vi "initiate.vi"(8 "error in (no error)":errorcluster, 11 "reference in":refnum<class "Devices Controller.lvclass">) -> (0 "error out":errorcluster, 3 "reference out":refnum<class "Devices Controller.lvclass">)   [LabVIEW 2016, in "Devices Controller.lvclass"]
uses:
  Devices Controller.lvclass
  File Controller_llb/File Controller.lvclass
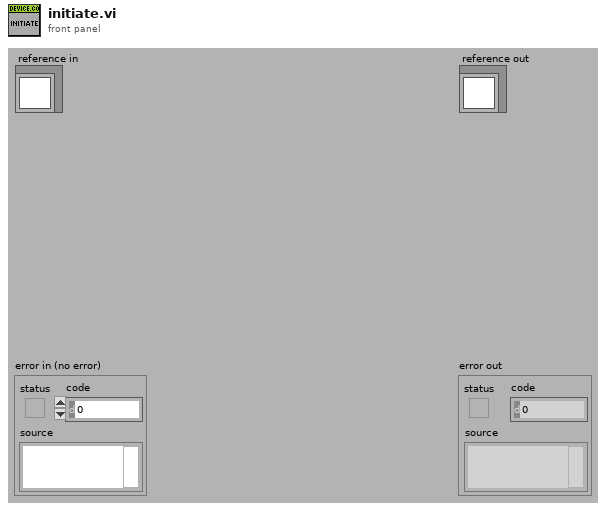
[diagram p1: front panel]
types:
  T1 = typedef "Devices Controller.lvclass/ObjectAttributesRef.ctl" = refnum<data-value>
  T2 = typedef "Devices Controller.lvclass/ObjectAttributes.ctl" = cluster{"MyAttribute":dbl, "file_controller_ref":refnum<class "File Controller.lvclass">, "data":string[][][], "devices_refs":cluster{"k4b2_refs":refnum<class "k4b2.lvclass">[], "rmr_refs":refnum<class "rmr.lvclass">[], "bod_pod_refs":refnum<class "bodpod.lvclass">[], "cpet_refs":refnum<class "cpet.lvclass">[], "fitmate_refs":refnum<class "fitmate.lvclass">[], "pea_pod_refs":refnum<class "peapod.lvclass">[], "k5_refs":refnum<class "k5.lvclass">[], "bb-pft_refs":refnum<class "bb-pft.lvclass">[]}}
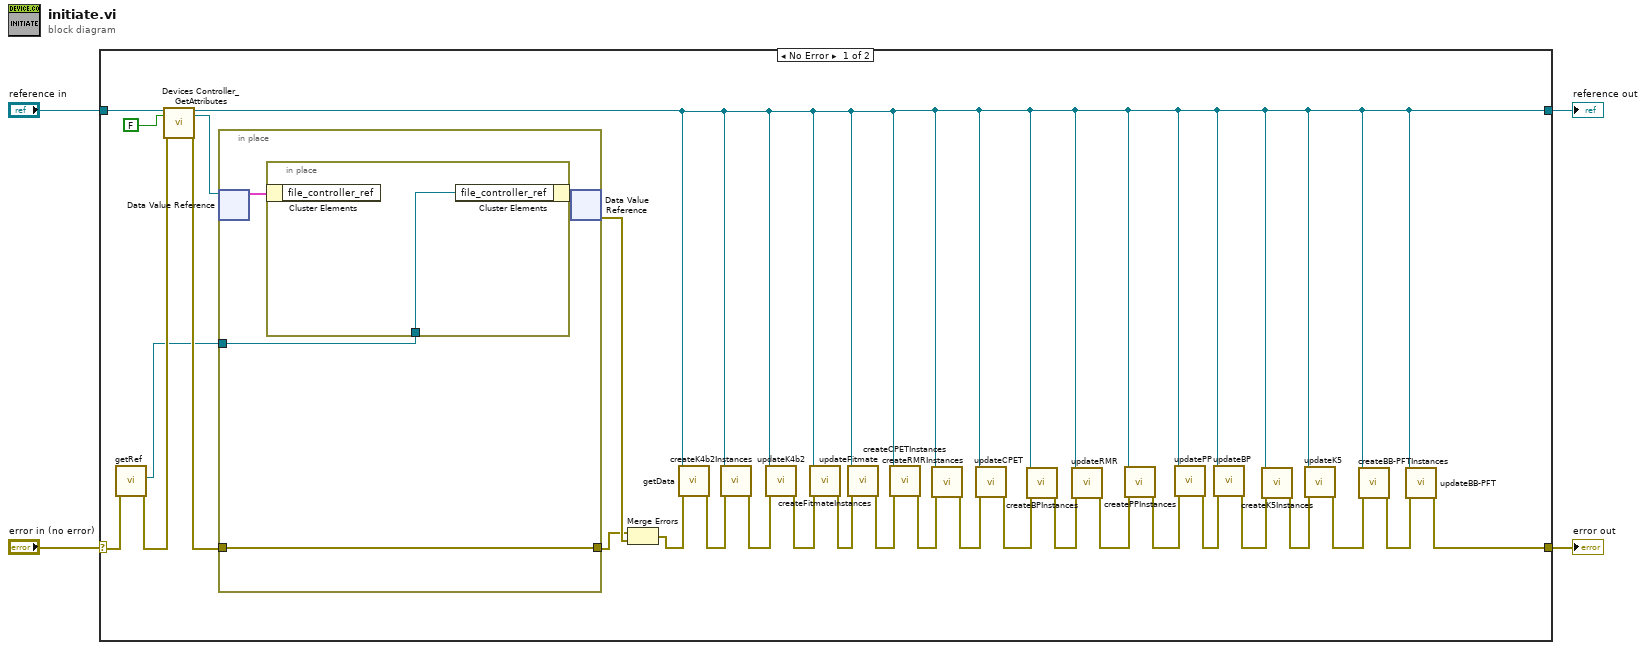
[diagram p0: block diagram]
diagram:
  n1 = case shown="No Error" "error in (no error)" {
    selector: "error in (no error)" -> [w13 w39]
    tunnel: [w5 w39] -> w3
    tunnel: [w8 w38] -> w1
    tunnel: "reference in" -> [w30 w38]
    frame No Error {
      n2 = call "getRef.vi"("error in (no error)"=w13) -> ("error out"=w12:errorcluster, "File Controller_ref"=w11:refnum<class "File Controller.lvclass">)  [unwired: 9 in]
      n3 = call "Devices Controller_GetAttributes.vi"("reference in"=w30, "return data? (T)"=FALSE, "error in (no error)"=w12) -> ("reference out"=w8:refnum<class "Devices Controller.lvclass">, "attributes ref"=w28:T1, "error out"=w27:errorcluster)  [unwired: 13 in, 1 out]
      n4 = in-place {
        in-place-border: w27 -> [w34]
        in-place-border: [w34] -> w31
        in-place-border: w11 -> [w33]
        n5 = in-place-dvr #1(w28) -> (w35:T2)  [unwired: 1 out]
        n6 = in-place {
          in-place-border: w33 -> [w37]
          n7 = in-place-cluster #2(w35) -> ()  [unwired: 1 out]
          n8 = in-place-cluster #2("file_controller_ref"=w37) -> (w36:T2)
        }
        n9 = in-place-dvr #1(w36) -> (w32:errorcluster)  [unwired: 1 out]
      }
      n10 = Merge Errors(w31, w32) -> (w26:errorcluster)
      n11 = call "getData.vi"("error in (no error)"=w26, "reference in"=w8) -> ("error out"=w25:errorcluster)  [unwired: 7 in, 2 out]
      n12 = call "createK4b2Instances.vi"("error in (no error)"=w25, "reference in"=w8) -> ("error out"=w23:errorcluster)  [unwired: 8 in, 1 out]
      n13 = call "updateK4b2.vi"("error in (no error)"=w23, "reference in"=w8) -> ("error out"=w22:errorcluster)  [unwired: 8 in, 1 out]
      n14 = call "createFitmateInstances.vi"("error in (no error)"=w22, "reference in"=w8) -> ("error out"=w21:errorcluster)  [unwired: 8 in, 1 out]
      n15 = call "updateFitmate.vi"("error in (no error)"=w21, "reference in"=w8) -> ("error out"=w20:errorcluster)  [unwired: 8 in, 1 out]
      n16 = call "createCPETInstances.vi"("error in (no error)"=w20, "reference in"=w8) -> ("error out"=w24:errorcluster)  [unwired: 8 in, 1 out]
      n17 = call "createRMRInstances.vi"("error in (no error)"=w24, "reference in"=w8) -> ("error out"=w19:errorcluster)  [unwired: 8 in, 1 out]
      n18 = call "updateCPET.vi"("error in (no error)"=w19, "reference in"=w8) -> ("error out"=w18:errorcluster)  [unwired: 8 in, 1 out]
      n19 = call "createBPInstances.vi"("error in (no error)"=w18, "reference in"=w8) -> ("error out"=w17:errorcluster)  [unwired: 8 in, 1 out]
      n20 = call "updateRMR.vi"("error in (no error)"=w17, "reference in"=w8) -> ("error out"=w16:errorcluster)  [unwired: 8 in, 1 out]
      n21 = call "createPPInstances.vi"("error in (no error)"=w16, "reference in"=w8) -> ("error out"=w15:errorcluster)  [unwired: 8 in, 1 out]
      n22 = call "updatePP.vi"("error in (no error)"=w15, "reference in"=w8) -> ("error out"=w14:errorcluster)  [unwired: 8 in, 1 out]
      n23 = call "updateBP.vi"("error in (no error)"=w14, "reference in"=w8) -> ("error out"=w10:errorcluster)  [unwired: 8 in, 1 out]
      n24 = call "createK5Instances.vi"("error in (no error)"=w10, "reference in"=w8) -> ("error out"=w9:errorcluster)  [unwired: 8 in, 1 out]
      n25 = call "updateK5.vi"("error in (no error)"=w9, "reference in"=w8) -> ("error out"=w7:errorcluster)  [unwired: 8 in, 1 out]
      n26 = call "createBB-PFTInstances.vi"("error in (no error)"=w7, "reference in"=w8) -> ("error out"=w6:errorcluster)  [unwired: 8 in, 1 out]
      n27 = call "updateBB-PFT.vi"("error in (no error)"=w6, "reference in"=w8) -> ("error out"=w5:errorcluster)  [unwired: 8 in, 1 out]
    }
    frame Error {
    }
  }
  "error out" <- w3
  "reference out" <- w1
